vi "VI CAN Konfig.vi"() -> ()   [LabVIEW 2020, in "CAN Konfig.lvlib"]
uses:
  CAN Konfig.lvlib
  Konfig Daten PC.ctl
  cRIO/CAN Interface/Baude Rate.ctl
  Visualisierungs Elemente/Button.ctl
  Aktion FGV CAN.ctl
  FT-IR/FGV FT-IR Gasliste Aktionen.ctl
  Passwortverwaltung/FGV Passwort Aktion.ctl
  Aktion Tabellen ziehen.ctl
  Allgemein/Aktionen Daten am cRIO speichern.ctl
  FT-IR/FGV FT-IR Aktionen.ctl
  SysLog/SysLog Interface.ctl
  Visualisierungs Elemente/String - Ausgabefeld.ctl
  Allgemein/allgemeine Sub-VIs.lvlib
  FT-IR/FT-IR.lvlib
  Sprachverwaltung/Sprachverwaltung.lvlib
  SysLog/SysLog.lvlib
  Passwortverwaltung/Passwort.lvlib
  cRIO/CAN Interface/CAN Interface.lvlib
panel:
  in  "exportieren":T1 caption="speichern"
  out "Status":u32[](array[numeric])
  in  "laden":T1 caption="speichern"
  in  "Konfig Daten":T2={"Baude Rate"=250000, "COM state"=0, "Frame-ID FTIR Start"=0, "Frame-ID FTIR End"=0, "Frame-ID Status Start"=0, "Frame-ID Status End"=0, "Zustand Information"=0, "Aktion"=0, "Frame-ID FTIR Arry"=[], "Frame-ID Status Arry"=[], "GPS Start"=0, "Interface"="CAN1"} {"Baude Rate" items=["40 kBaud"=40000, "50 kBaud"=50000, "62,5 kBaud"=62500, "80 kBaud"=80000, "83,3 kBaud"=83300, "100 kBaud"=100000, "125 kBaud"=125000, "160 kBaud"=160000, "200 kBaud"=200000, "250 kBaud"=250000, "400 kBaud"=400000, "500 kBaud"=500000, "800 kBaud"=800000, "1 MBaud"=1000000]}
  in  "Optionsfelder FT-IR":T4(radio)
  in  "Optionsfelder Status":T4(radio)
  in  "Tabellenelement FT-IR":string[][](table)
  in  "Tabellenelement Status":string[][](table)
  in  "Löschen Status":bool
  in  "Entfernen Status":bool
  in  "Hinzufügen Status":bool
  in  "Konfigurierte Liste Status":i32(listbox)=-1 caption="Konfigurierte Liste"
  in  "Statusliste":i32(listbox)=-1 caption="Original Liste"
  in  "Löschen FTIR 1":bool
  in  "Entfernen FTIR 1":bool
  in  "Hinzufügen FTIR 1":bool
  in  "speichern":T1
  in  "Konfigurierte Liste 1":i32(listbox)=-1 caption="Konfigurierte Liste"
  in  "Original Liste":i32(listbox)=-1
  in  "apply":T1 caption="speichern"
  # "CAN Config"
  # "Scale"
  # "Scale"
  # "CAN Parameter"
  # "Status Frame"
  # "Status Value"
  # "FTIR Frame"
  # "Gaslist"
  # "CAN Measurement Data"
  # "CAN Status Value"
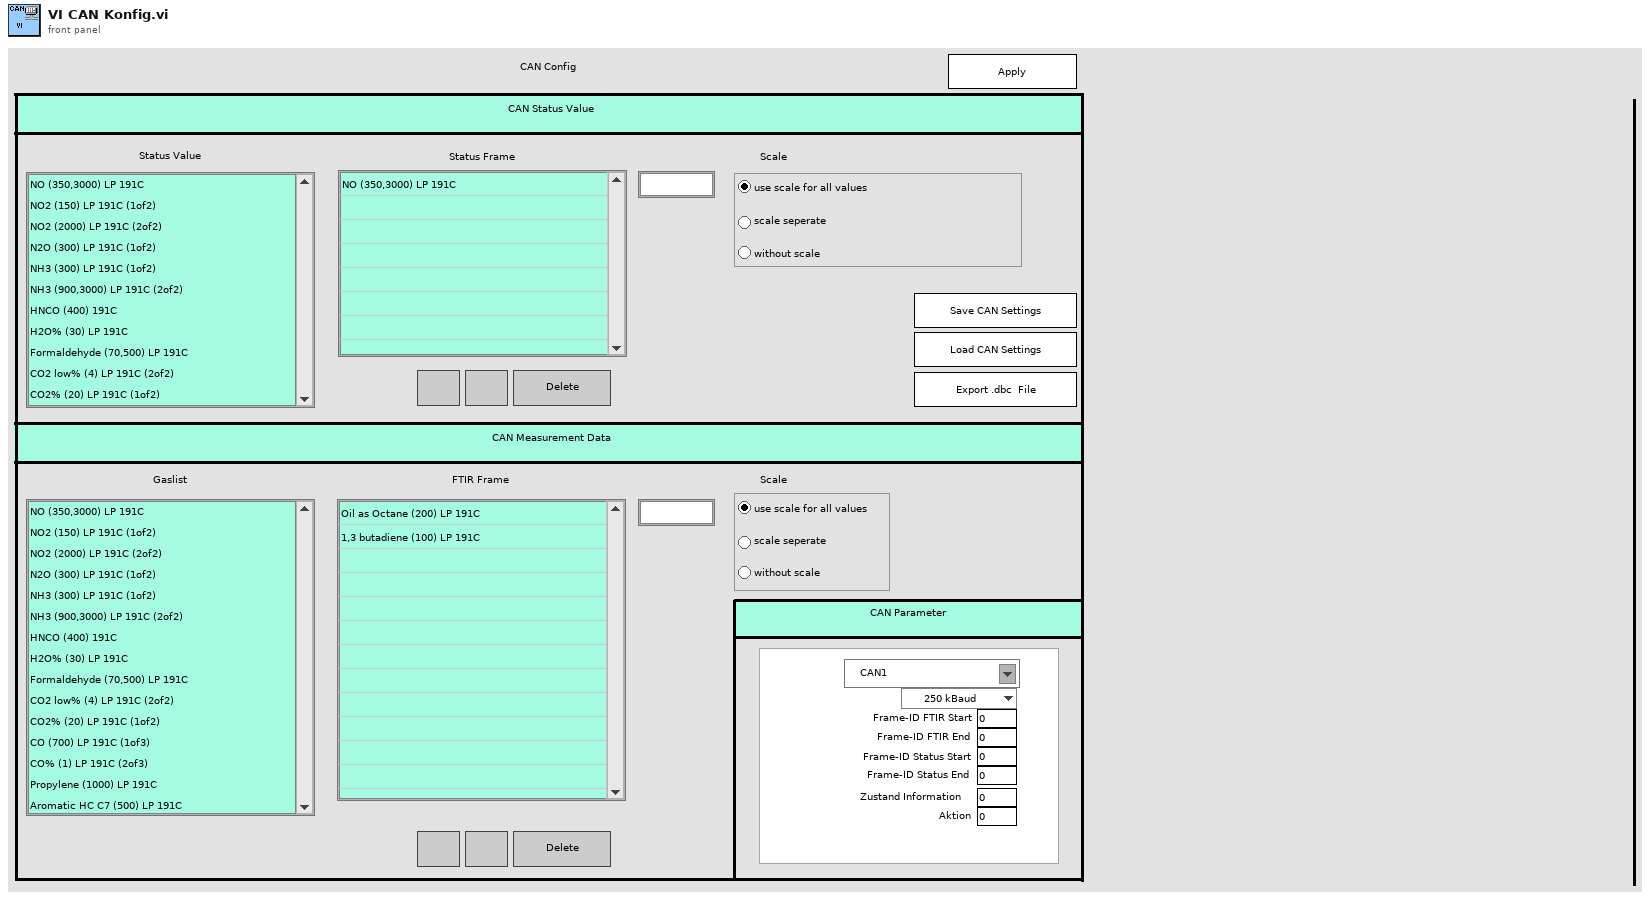
[diagram p1: front panel]
types:
  T1 = typedef "Button.ctl" = bool
  T2 = typedef "CAN Konfig.lvlib/Konfig Daten PC.ctl" = cluster{"Baude Rate":T3, "COM state":u8, "Frame-ID FTIR Start":u32, "Frame-ID FTIR End":u32, "Frame-ID Status Start":u32, "Frame-ID Status End":u32, "Zustand Information":u32, "Aktion":u32, "Frame-ID FTIR Arry":u32[], "Frame-ID Status Arry":u32[], "GPS Start":u32, "Interface":refnum<k21>}
  T3 = typedef "CAN Interface.lvlib/Baude Rate.ctl" = u32
  T4 = enum32{"Optionsauswahl 1", "Optionsauswahl 2", "Optionsauswahl 3"}
  T5 = typedef "Passwort.lvlib/FGV Passwort Aktion.ctl" = enum16{"prüfen", "setzen", "Initialisieren", "PW speichern", "lesen", "PW Änderung"}
  T6 = typedef "FT-IR.lvlib/FGV FT-IR Gasliste Aktionen.ctl" = enum16{"lesen", "Gasliste FT-IR", "Gasliste ausgelesen", "laden", "speichern", "löschen"}
  T7 = typedef "CAN Konfig.lvlib/Aktion FGV CAN.ctl" = enum16{"lesen", "schreiben Konfig", "Status", "Messdaten", "laden", "speichern", "CAN Data"}
  T8 = typedef "CAN Konfig.lvlib/Aktion Tabellen ziehen.ctl" = enum16{"ini", "prüfen"}
  T9 = typedef "CAN Konfig.lvlib/CAN Messdaten.ctl" = cluster{"FTIR 1 Index":i32[], "FTIR 2 Index":i32[], "Status Index":i32[], "FT-IR Scale":sgl[], "Status Scale":sgl[], "Optionsfelder FT-IR":enum32{"Optionsauswahl 1", "Optionsauswahl 2", "Optionsauswahl 3"}, "Optionsfelder Status":enum32{"Optionsauswahl 1", "Optionsauswahl 2", "Optionsauswahl 3"}}
  T10 = typedef "String - Ausgabefeld.ctl" = string
  T11 = typedef "allgemeine Sub-VIs.lvlib/Aktionen Daten am cRIO speichern.ctl" = enum16{"lesen", "speichern setzen", "speichern reset", "gespeichert"}
  T12 = typedef "FT-IR.lvlib/FGV FT-IR Aktionen.ctl" = enum16{"lesen", "NOG setzen", "NOS setzen", "Initialisieren", "speichern", "ALLES setzen", "FT-IR Spektrum loggen", "Komm Stoppen", "Spektrum LogKonfig"}
  T13 = typedef "SysLog.lvlib/SysLog Interface.ctl" = cluster{"FehlermeldungsCode":i32, "ErfolgsmeldungsCode":i32, "ParameterListenString":string, "Anzeige":bool, "SysLogIcon":enum16{"OK", "Warnung", "Fehler"}, "intern":bool}
  T14 = enum16{"Left Button", "Center Button", "Right Button", "Window Close"}
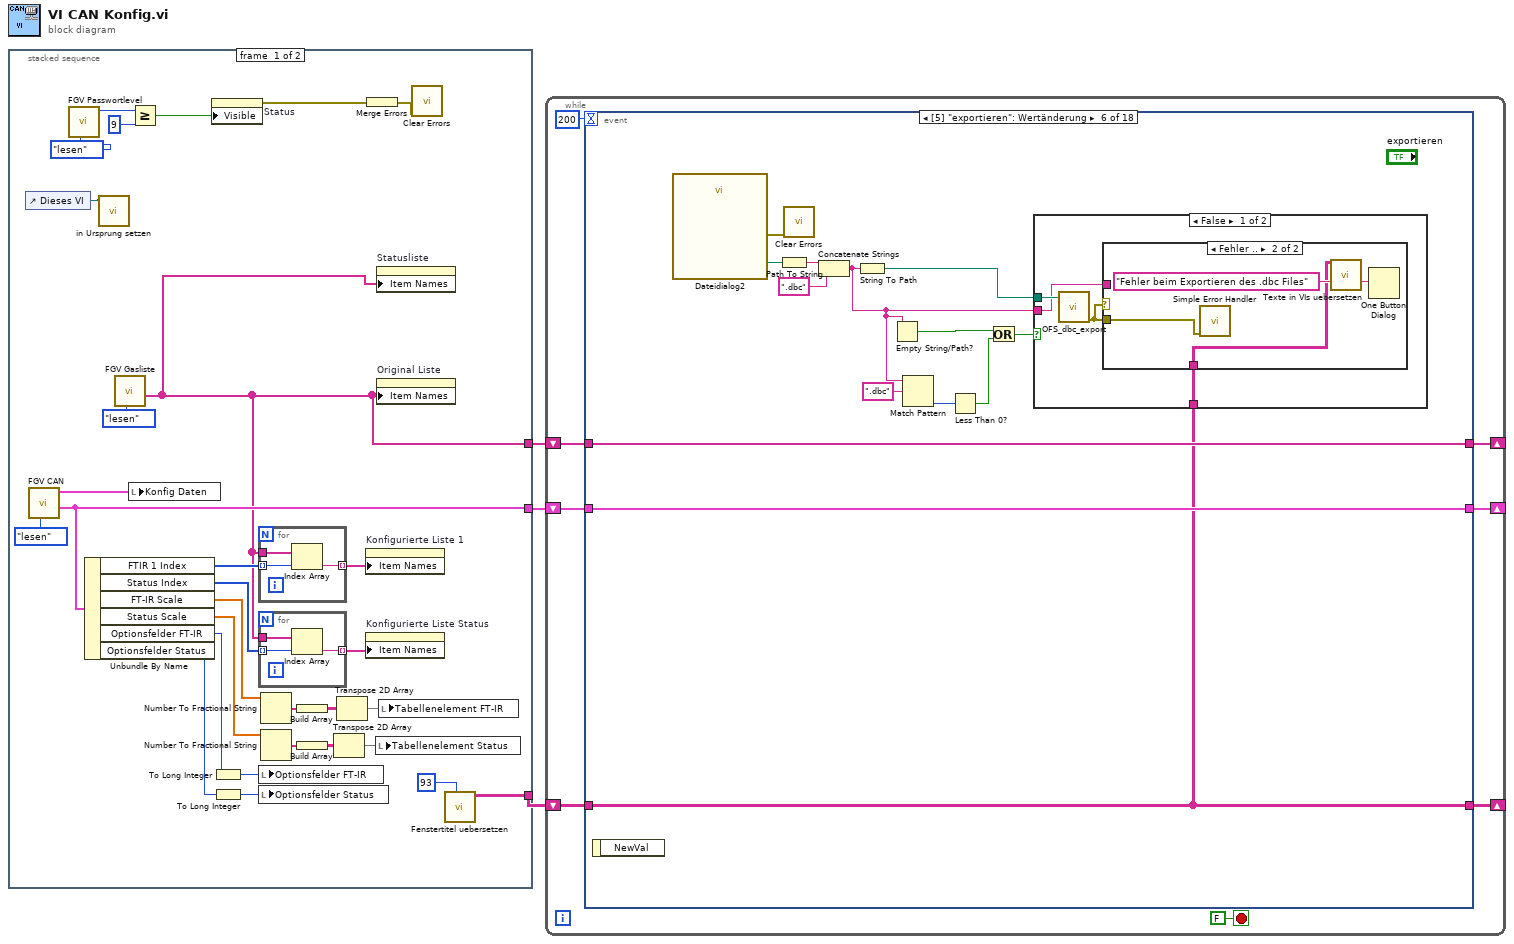
[diagram p0: block diagram]
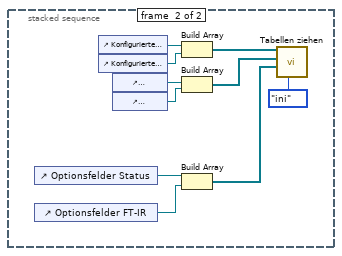
[diagram p2: hidden frame]
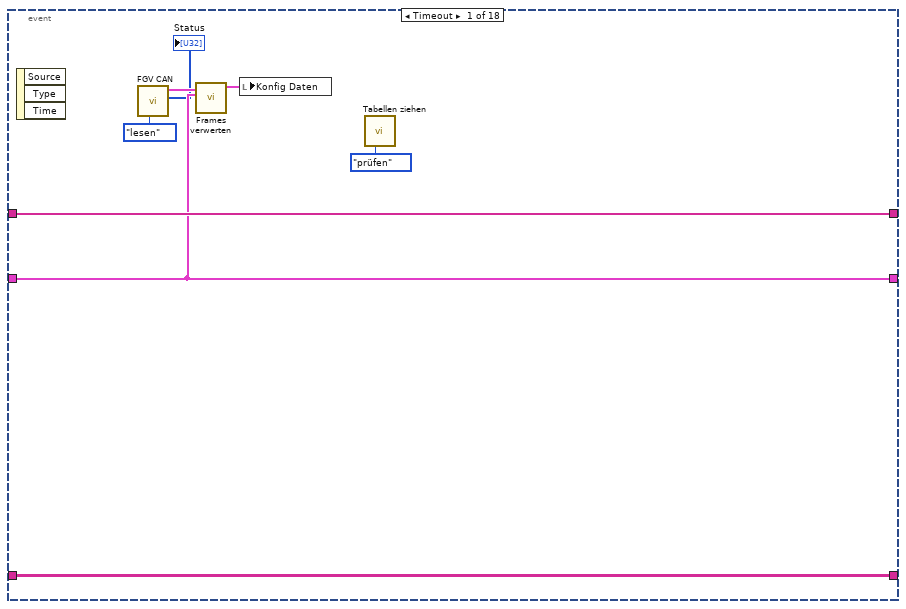
[diagram p3: hidden frame]
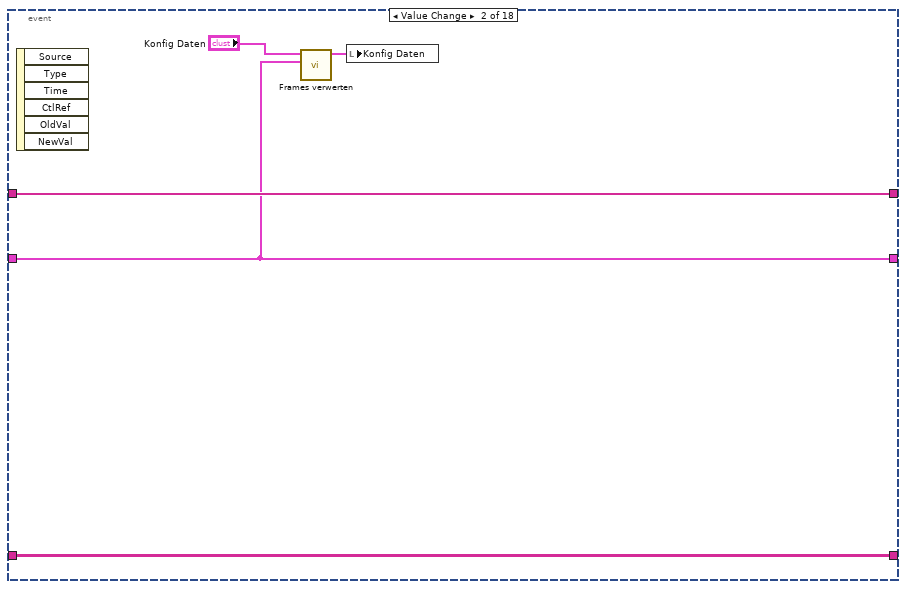
[diagram p4: hidden frame]
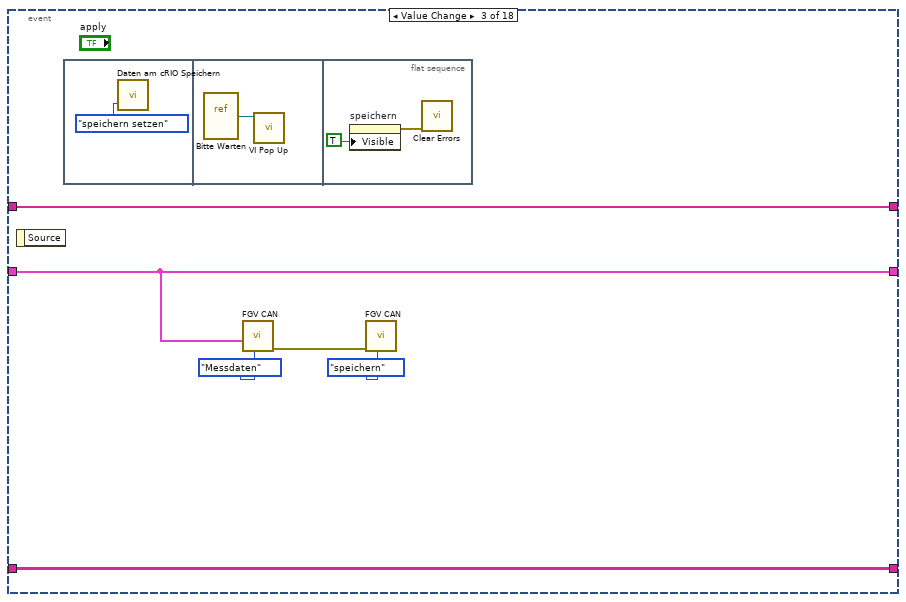
[diagram p5: hidden frame]
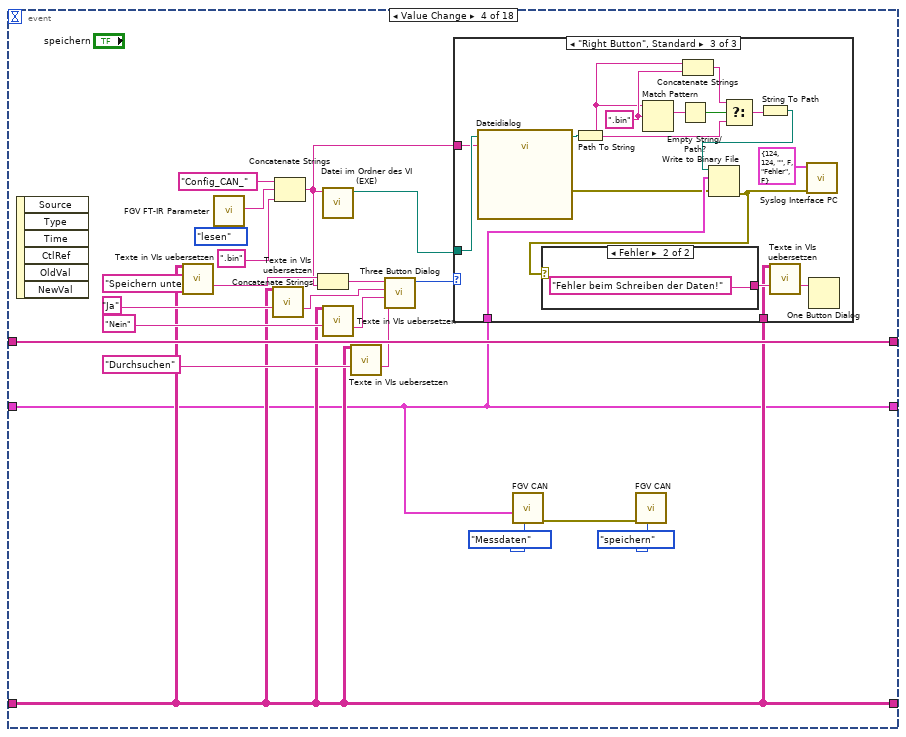
[diagram p6: hidden frame]
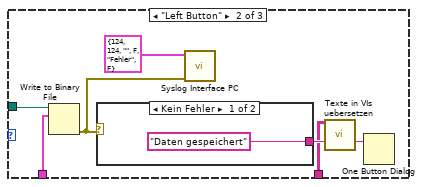
[diagram p8: hidden frame]
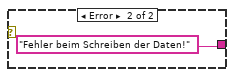
[diagram p9: hidden frame]
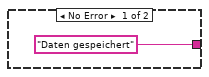
[diagram p10: hidden frame]
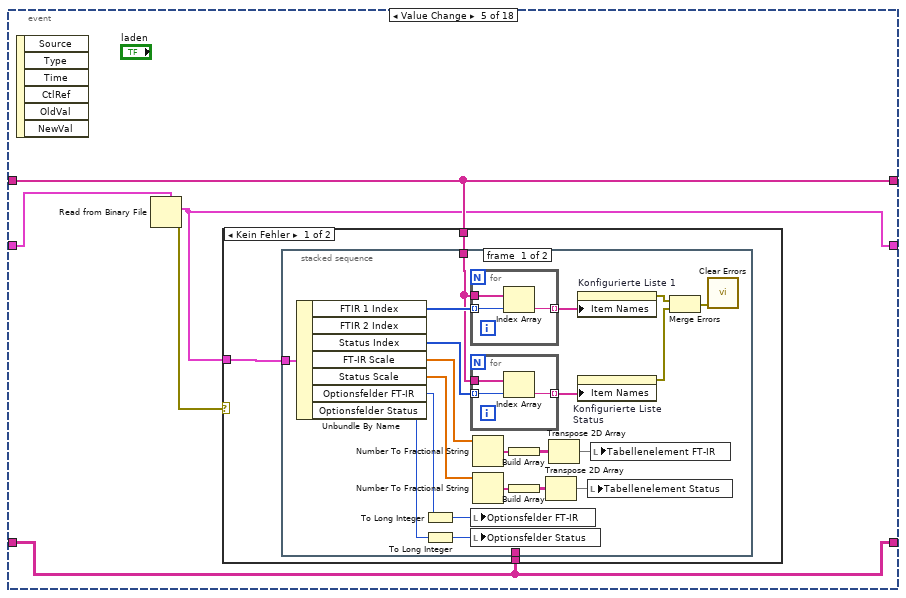
[diagram p11: hidden frame]
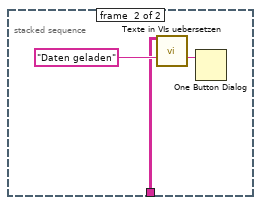
[diagram p12: hidden frame]
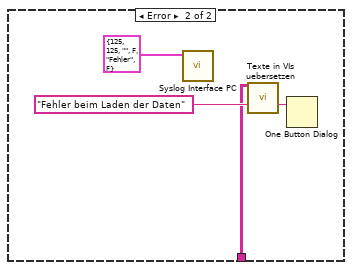
[diagram p13: hidden frame]
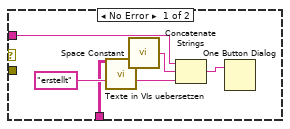
[diagram p14: hidden frame]
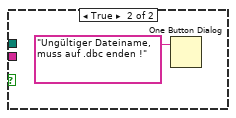
[diagram p15: hidden frame]
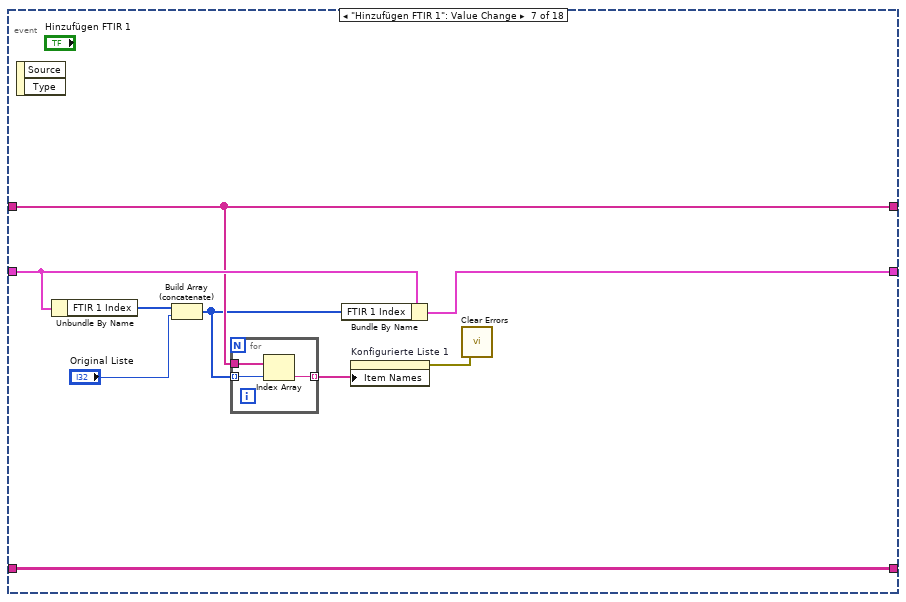
[diagram p16: hidden frame]
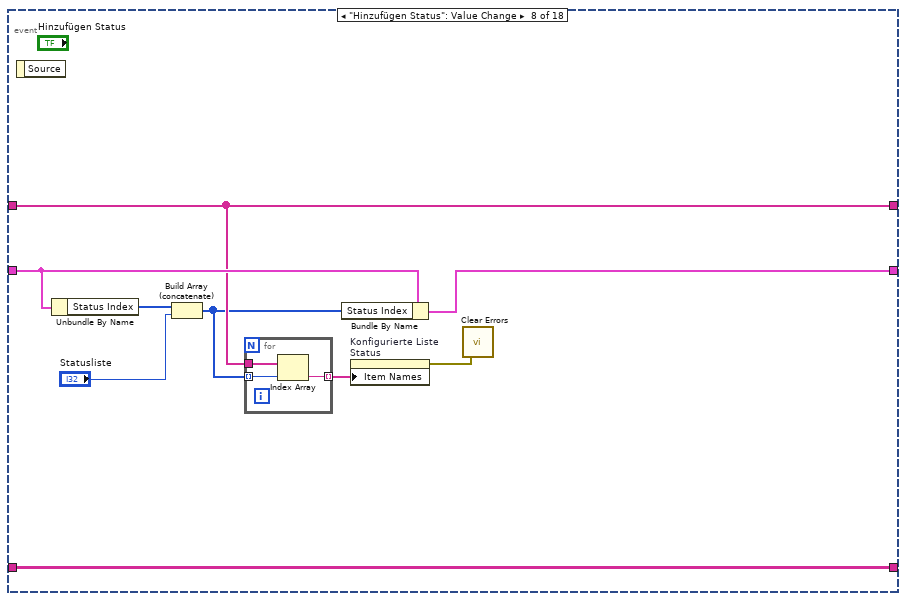
[diagram p17: hidden frame]
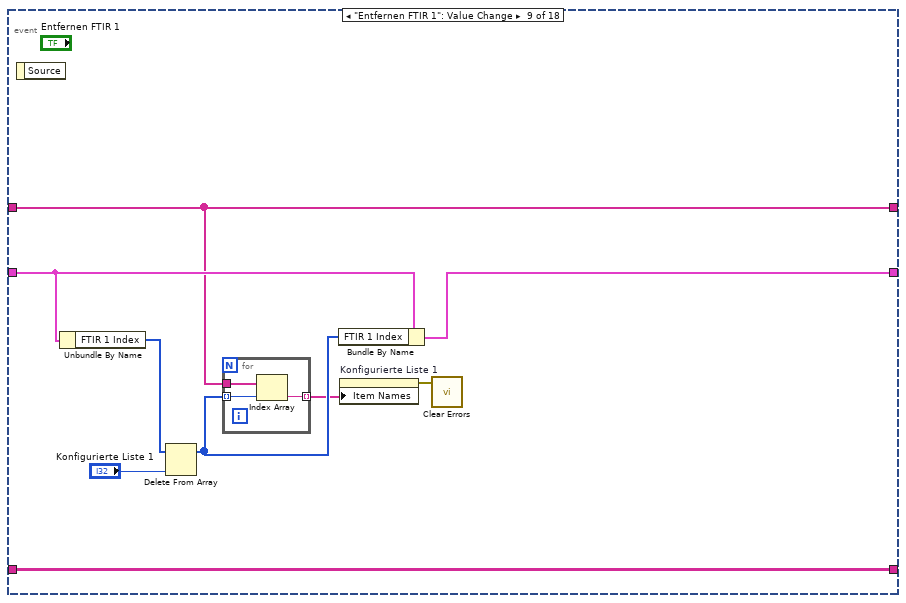
[diagram p18: hidden frame]
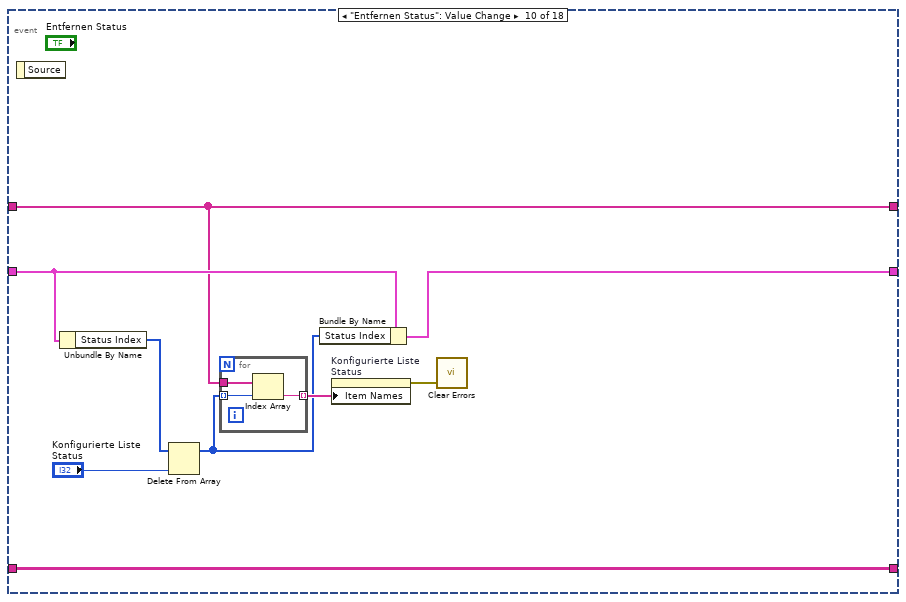
[diagram p19: hidden frame]
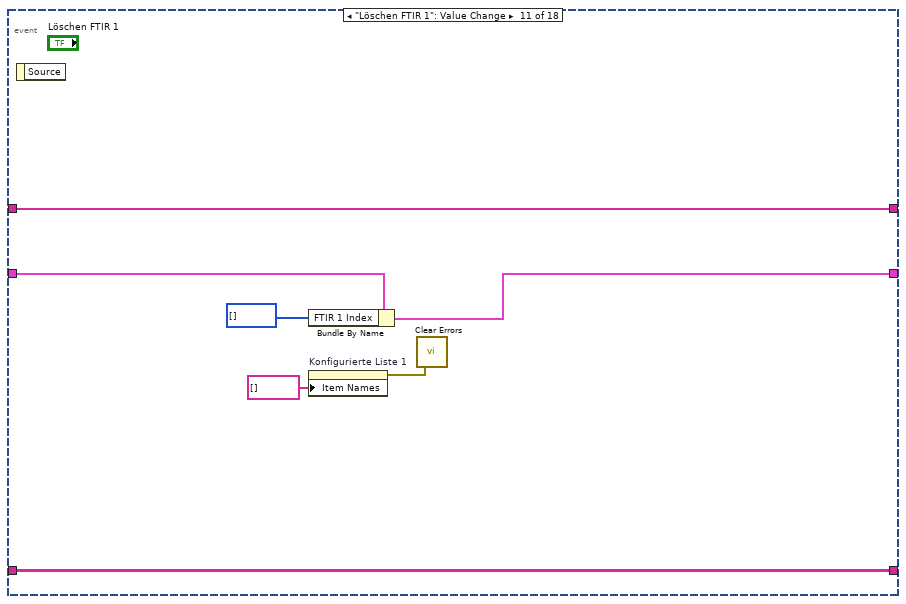
[diagram p20: hidden frame]
diagram:
  n1 = stacked-sequence {
    tunnel: [w4 _] -> w3
    tunnel: [w29 _] -> w2
    tunnel: [w11 _] -> w1
    frame #0 {
      n2 = control-ref of="Dieses VI"() -> (w25:refnum<vi>)
      n3 = call "FGV CAN.vi"("Aktion"=Aktion_FGV_CAN."lesen") -> ("CAN Messdaten"=w29:T9, "Konfig Daten"=w32:T2)  [unwired: 6 in, 3 out]
      n4 = call "FGV Passwortlevel.vi"("FGV Passwort Aktion"=FGV_Passwort_Aktion."lesen") -> ("aktueller Level"=w8:i16)  [unwired: 8 in, 2 out]
      n5 = Unbundle By Name(w29) -> ("FTIR 1 Index"=w30:i32[], "Status Index"=w27:i32[], "FT-IR Scale"=w24:sgl[], "Status Scale"=w23:sgl[], "Optionsfelder FT-IR"=w18:T4, "Optionsfelder Status"=w16:T4)
      n6 = call "in Ursprung setzen.vi"("VI Referenz"=w25) -> ()  [unwired: 10 in, 1 out]
      n7 = call "FGV Gasliste.vi"("Aktionen"=FGV_FT-IR_Gasliste_Aktionen."lesen") -> ("Aktuelle Gasliste gesamt"=w4:T10[])  [unwired: 8 in, 2 out]
      n8 = local write "Konfig Daten"(w32) -> ()
      n9 = Greater Or Equal?(x=w8, y=i16 9 ("x")) -> (x >= y?=w7:bool)
      n10 = property on="Status" class="Arr (strikt)"("Visible"=w7) -> (error out=w6:errorcluster)  [unwired: 2 in, 1 out]
      n11 = To Long Integer(number=w18) -> (32bit integer=w17:i32)
      n12 = To Long Integer(number=w16) -> (32bit integer=w15:i32)
      n13 = for {
        tunnel: w30 -> [w39] mode=indexing
        tunnel: w4 -> [w38]
        tunnel: [w37] -> w31 mode=indexing
        n14 = Index Array(array=w38, index=w39) -> (element=w37:T10)
      }
      n15 = for {
        tunnel: [w36] -> w28 mode=indexing
        tunnel: w27 -> [w35] mode=indexing
        tunnel: w4 -> [w34]
        n16 = Index Array(array=w34, index=w35) -> (element=w36:T10)
      }
      n17 = local write "Optionsfelder FT-IR"(w17) -> ()
      n18 = local write "Optionsfelder Status"(w15) -> ()
      n19 = Number To Fractional String(number=w24) -> (F-format string=w19:string[])  [unwired: 3 in]
      n20 = Number To Fractional String(number=w23) -> (F-format string=w22:string[])  [unwired: 3 in]
      n21 = Build Array(w19) -> (w20:string[][])
      n22 = Build Array(w22) -> (w21:string[][])
      n23 = Transpose 2D Array(2D array=w21) -> (transposed array=w13:string[][])
      n24 = Transpose 2D Array(2D array=w20) -> (transposed array=w14:string[][])
      n25 = property on="Konfigurierte Liste 1" class="Listenfeld (strikt)"("Item Names"=w31) -> ()  [unwired: 2 in, 2 out]
      n26 = property on="Konfigurierte Liste Status" class="Listenfeld (strikt)"("Item Names"=w28) -> ()  [unwired: 2 in, 2 out]
      n27 = Merge Errors(w6) -> (w5:errorcluster)
      n28 = local write "Tabellenelement Status"(w13) -> ()
      n29 = property on="Statusliste" class="Listenfeld (strikt)"("Item Names"=w4) -> ()  [unwired: 2 in, 2 out]
      n30 = property on="Original Liste" class="Listenfeld (strikt)"("Item Names"=w4) -> ()  [unwired: 2 in, 2 out]
      n31 = local write "Tabellenelement FT-IR"(w14) -> ()
      n32 = call <vilib>:"Clear Errors.vi"("error in (no error)"=w5) -> ()  [unwired: 5 in, 2 out]
      n33 = call "Fenstertitel uebersetzen.vi"("Index (Seite)"=93) -> ("Sprachliste"=w11:string[][])  [unwired: 7 in, 3 out]
    }
    frame #1 {
      n34 = control-ref of="Optionsfelder Status"() -> (w43:refnum<vi>)
      n35 = control-ref of="Optionsfelder FT-IR"() -> (w42:refnum<vi>)
      n36 = control-ref of="Konfigurierte Liste Status"() -> (w46:refnum<vi>)
      n37 = control-ref of="Konfigurierte Liste 1"() -> (w47:refnum<vi>)
      n38 = control-ref of="Tabellenelement Status"() -> (w48:refnum<vi>)
      n39 = control-ref of="Tabellenelement FT-IR"() -> (w49:refnum<vi>)
      n40 = Build Array(w46, w47) -> (w45:refnum<vi>[])
      n41 = Build Array(w48, w49) -> (w44:refnum<vi>[])
      n42 = Build Array(w43, w42) -> (w41:refnum<vi>[])
      n43 = call "Tabellen ziehen.vi"("Aktion"=Aktion_Tabellen_ziehen."ini", "Angehängtes Array"=w41, "Tabelle (Eingang)"=w44, "Konfigurierte Liste Status"=w45) -> ()  [unwired: 8 in]
    }
  }
  n44 = while {
    shift-right: [w55] -> _
    shift-left: w3 -> [w56]
    shift-right: [w53] -> _
    shift-left: w2 -> [w54]
    shift-right: [w50] -> _
    shift-left: w1 -> [w51]
    stop <- FALSE stop-if-true
    n45 = event shown="[5] \"exportieren\": Wertänderung" {
      selector: _ -> [_ _ _ _ _ _ _ _ _ _ _ _ _ _ _ _ _ _]
      dyn-events: _ -> [_ _ _ _ _ _ _ _ _ _ _ _ _ _ _ _ _ _]
      timeout: 200 -> [_ _ _ _ _ _ _ _ _ _ _ _ _ _ _ _ _ _]
      tunnel: w56 -> [w65 w70 w76 w102 w135 w186 w204 w215 w227 w239 w256 w263 w274 w304 w333 w343 w349 w360]
      tunnel: [w65 w70 w76 w102 w135 w186 w204 w215 w227 w239 w256 w263 w274 w304 w333 w343 w349 w360] -> w55
      tunnel: w54 -> [w61 w68 w72 w81 w134 w185 w209 w221 w234 w246 w255 w262 w270 w300 w327 w337 w348 w359]
      tunnel: [w61 w68 w72 w81 w133 w185 w208 w220 w231 w244 w254 w261 w273 w303 w325 w335 w345 w356] -> w53
      tunnel: w51 -> [w59 w66 w71 w87 w131 w173 w206 w217 w229 w241 w251 w257 w264 w294 w324 w334 w344 w355]
      tunnel: [w59 w66 w71 w87 w131 w173 w206 w217 w229 w241 w251 w257 w264 w294 w324 w334 w344 w355] -> w50
      event Timeout {
        n46 = event-data() -> ()  [unwired: 1 in, 3 out]
        n47 = call "FGV CAN.vi"("Aktion"=Aktion_FGV_CAN."lesen") -> ("Status"=→"Status":u32[], "Konfig Daten"=w62:T2)  [unwired: 6 in, 3 out]
        n48 = call "Frames verwerten.vi"("CAN Messdaten"=w61, "Konfig Daten"=w62) -> ("Ausgangs-Cluster"=w63:T2)  [unwired: 9 in]
        n49 = local write "Konfig Daten"(w63) -> ()
        n50 = call "Tabellen ziehen.vi"("Aktion"=Aktion_Tabellen_ziehen."prüfen") -> ()  [unwired: 11 in]
      }
      event Value Change {
        n51 = event-data() -> ()  [unwired: 1 in, 6 out]
        n52 = call "Frames verwerten.vi"("CAN Messdaten"=w68, "Konfig Daten"="Konfig Daten") -> ("Ausgangs-Cluster"=w67:T2)  [unwired: 9 in]
        n53 = local write "Konfig Daten"(w67) -> ()
      }
      event Value Change {
        n54 = event-data() -> ()  [unwired: 1 in, 1 out]
        n55 = flat-sequence {
          frame #0 {
            n56 = call "Daten am cRIO Speichern.vi"("Aktionen"=Aktionen_Daten_am_cRIO_speichern."speichern setzen") -> ()  [unwired: 9 in, 2 out]
          }
          frame #1 {
            n57 = vi-ref "Bitte Warten.vi"() -> (w78:refnum<vi>)
            n58 = call "VI Pop Up.vi"("VI Referenz"=w78) -> ()  [unwired: 10 in, 1 out]
          }
          frame #2 {
            n59 = property on="speichern" class="Bool."("Visible"=TRUE ("Sichtbar")) -> (error out=w79:errorcluster)  [unwired: 2 in, 1 out]
            n60 = call <vilib>:"Clear Errors.vi"("error in (no error)"=w79) -> ()  [unwired: 5 in, 2 out]
          }
        }
        n61 = call "FGV CAN.vi"("Aktion"=Aktion_FGV_CAN."Messdaten", "CAN Messdaten"=w72) -> ("error out"=w73:errorcluster)  [unwired: 5 in, 4 out]
        n62 = call "FGV CAN.vi"("Aktion"=Aktion_FGV_CAN."speichern", "error in (no error)"=w73) -> ()  [unwired: 5 in, 5 out]
      }
      event Value Change {
        n63 = event-data() -> ()  [unwired: 1 in, 6 out]
        n64 = call "Texte in VIs uebersetzen.vi"("Sprachliste"=w87, "String zum Übersetzen"="Speichern unter ") -> ("String zum Übersetzen"=w91:string)  [unwired: 9 in, 4 out]
        n65 = call "FGV FT-IR Parameter.vi"("Aktion"=FGV_FT-IR_Aktionen."lesen") -> ("Current Recipe"=w99:string)  [unwired: 11 in, 7 out]
        n66 = call "Texte in VIs uebersetzen.vi"("Sprachliste"=w87, "String zum Übersetzen"="Ja") -> ("String zum Übersetzen"=w90:string)  [unwired: 9 in, 4 out]
        n67 = Concatenate Strings("Config_CAN_" ("Dateiname"), w99, ".bin" ("Dateiname")) -> (w85:string)
        n68 = Concatenate Strings(w91, w85) -> (w96:string)
        n69 = call "Datei im Ordner des VI (EXE).vi"("Dateiname"=w85) -> ("Dateipfad im Ordner des Haupt-VIs"=w97:path)  [unwired: 8 in, 2 out]
        n70 = call "Texte in VIs uebersetzen.vi"("Sprachliste"=w87, "String zum Übersetzen"="Nein") -> ("String zum Übersetzen"=w89:string)  [unwired: 9 in, 4 out]
        n71 = call "Texte in VIs uebersetzen.vi"("Sprachliste"=w87, "String zum Übersetzen"="Durchsuchen") -> ("String zum Übersetzen"=w86:string)  [unwired: 9 in, 4 out]
        n72 = call <vilib>:"Three Button Dialog.vi"("Right Button Text (\"Cancel\")"=w86, "Center Button Text (\"No\")"=w89, "Left Button Text (\"Yes\")"=w90, "message"=w96) -> ("Which Button?"=w95:T14)  [unwired: 7 in]
        n73 = case shown="\"Right Button\", Standard" w95 {
          tunnel: w97 -> [_ w109 w125]
          tunnel: w81 -> [_ w108 w123]
          tunnel: w87 -> [_ w105 w126]
          tunnel: w85 -> [_ _ w124]
          frame "Center Button" {
          }
          frame "Left Button" {
            n74 = Write to Binary File(file (use dialog)=w109, data=w108) -> (error out=w103:errorcluster)  [unwired: 1 in, 5 out]
            n75 = case shown="Kein Fehler" w103 {
              tunnel: ["Daten gespeichert" ("String") "Fehler beim Schreiben der Daten!" ("String")] -> w107
              frame No Error {
              }
              frame Error {
              }
            }
            n76 = call "Syslog Interface PC.vi"("Fehler (in)"=w103, "Cluster (in)"=T13 {"FehlermeldungsCode"=124, "ErfolgsmeldungsCode"=124, "ParameterListenString"="", "Anzeige"=FALSE, "SysLogIcon"=enum."Fehler", "intern"=FALSE}) -> ()  [unwired: 9 in, 1 out]
            n77 = call "Texte in VIs uebersetzen.vi"("Sprachliste"=w105, "String zum Übersetzen"=w107) -> ("String zum Übersetzen"=w106:string)  [unwired: 9 in, 4 out]
            n78 = One Button Dialog(message=w106) -> ()  [unwired: 1 in, 1 out]
          }
          frame "Right Button", Default {
            w115 = ".bin" ("Regulärer Ausdruck")
            n79 = call "Dateidialog"("start path"=w125, "default name"=w124) -> ("selected path"=w120:path, "error out"=w118:errorcluster)  [unwired: 10 in, 2 out]
            n80 = Path To String(path=w120) -> (string=w113:string)
            n81 = Match Pattern(string=w113, regular expression=w115) -> (match substring=w116:string)  [unwired: 1 in, 3 out]
            n82 = Empty String/Path?(string/path=w116) -> (empty?=w117:bool)
            n83 = Concatenate Strings(w113, w115) -> (w114:string)
            n84 = Select(t=w114, s=w117, f=w113) -> (s? t:f=w112:string)
            n85 = String To Path(string=w112) -> (path=w119:path)
            n86 = Write to Binary File(file (use dialog)=w119, data=w123, error in=w118) -> (error out=w121:errorcluster)  [unwired: 5 out]
            n87 = case shown="Fehler" w121 {
              tunnel: ["Daten gespeichert" ("String") "Fehler beim Schreiben der Daten!" ("String")] -> w128
              frame No Error {
              }
              frame Error {
              }
            }
            n88 = call "Texte in VIs uebersetzen.vi"("Sprachliste"=w126, "String zum Übersetzen"=w128) -> ("String zum Übersetzen"=w127:string)  [unwired: 9 in, 4 out]
            n89 = call "Syslog Interface PC.vi"("Fehler (in)"=w121, "Cluster (in)"=T13 {"FehlermeldungsCode"=124, "ErfolgsmeldungsCode"=124, "ParameterListenString"="", "Anzeige"=FALSE, "SysLogIcon"=enum."Fehler", "intern"=FALSE}) -> ()  [unwired: 9 in, 1 out]
            n90 = One Button Dialog(message=w127) -> ()  [unwired: 1 in, 1 out]
          }
        }
        n91 = call "FGV CAN.vi"("Aktion"=Aktion_FGV_CAN."Messdaten", "CAN Messdaten"=w81) -> ("error out"=w82:errorcluster)  [unwired: 5 in, 4 out]
        n92 = call "FGV CAN.vi"("Aktion"=Aktion_FGV_CAN."speichern", "error in (no error)"=w82) -> ()  [unwired: 5 in, 5 out]
      }
      event Value Change {
        n93 = event-data() -> ()  [unwired: 1 in, 6 out]
        n94 = Read from Binary File(5:w134) -> (0:w132:errorcluster, 2:w133:T9)  [unwired: 2 in, 5 out]
        n95 = case shown="Kein Fehler" w132 {
          tunnel: w135 -> [w138 _]
          tunnel: w133 -> [w137 _]
          tunnel: w131 -> [w136 w170]
          frame No Error {
            n96 = stacked-sequence {
              tunnel: w138 -> [w143 _]
              tunnel: w137 -> [w142 _]
              tunnel: w136 -> [_ w166]
              frame #0 {
                n97 = Unbundle By Name(w142) -> ("FTIR 1 Index"=w145:i32[], "Status Index"=w147:i32[], "FT-IR Scale"=w148:sgl[], "Status Scale"=w149:sgl[], "Optionsfelder FT-IR"=w154:T4, "Optionsfelder Status"=w156:T4)  [unwired: 1 out]
                n98 = To Long Integer(number=w154) -> (32bit integer=w155:i32)
                n99 = To Long Integer(number=w156) -> (32bit integer=w157:i32)
                n100 = for {
                  tunnel: w145 -> [w165] mode=indexing
                  tunnel: w143 -> [w164]
                  tunnel: [w163] -> w144 mode=indexing
                  n101 = Index Array(array=w164, index=w165) -> (element=w163:T10)
                }
                n102 = for {
                  tunnel: [w162] -> w146 mode=indexing
                  tunnel: w147 -> [w161] mode=indexing
                  tunnel: w143 -> [w160]
                  n103 = Index Array(array=w160, index=w161) -> (element=w162:T10)
                }
                n104 = local write "Optionsfelder FT-IR"(w155) -> ()
                n105 = local write "Optionsfelder Status"(w157) -> ()
                n106 = Number To Fractional String(number=w148) -> (F-format string=w153:string[])  [unwired: 3 in]
                n107 = Number To Fractional String(number=w149) -> (F-format string=w150:string[])  [unwired: 3 in]
                n108 = Build Array(w153) -> (w152:string[][])
                n109 = Build Array(w150) -> (w151:string[][])
                n110 = Transpose 2D Array(2D array=w151) -> (transposed array=w159:string[][])
                n111 = Transpose 2D Array(2D array=w152) -> (transposed array=w158:string[][])
                n112 = property on="Konfigurierte Liste 1" class="Listenfeld (strikt)"("Item Names"=w144) -> (error out=w140:errorcluster)  [unwired: 2 in, 1 out]
                n113 = property on="Konfigurierte Liste Status" class="Listenfeld (strikt)"("Item Names"=w146) -> (error out=w139:errorcluster)  [unwired: 2 in, 1 out]
                n114 = local write "Tabellenelement Status"(w159) -> ()
                n115 = local write "Tabellenelement FT-IR"(w158) -> ()
                n116 = Merge Errors(w140, w139) -> (w141:errorcluster)
                n117 = call <vilib>:"Clear Errors.vi"("error in (no error)"=w141) -> ()  [unwired: 5 in, 2 out]
              }
              frame #1 {
                n118 = call "Texte in VIs uebersetzen.vi"("Sprachliste"=w166, "String zum Übersetzen"="Daten geladen" ("String")) -> ("String zum Übersetzen"=w168:string)  [unwired: 9 in, 4 out]
                n119 = One Button Dialog(message=w168) -> ()  [unwired: 1 in, 1 out]
              }
            }
          }
          frame Error {
            n120 = call "Syslog Interface PC.vi"("Cluster (in)"=T13 {"FehlermeldungsCode"=125, "ErfolgsmeldungsCode"=125, "ParameterListenString"="", "Anzeige"=FALSE, "SysLogIcon"=enum."Fehler", "intern"=FALSE}) -> ()  [unwired: 10 in, 1 out]
            n121 = call "Texte in VIs uebersetzen.vi"("Sprachliste"=w170, "String zum Übersetzen"="Fehler beim Laden der Daten" ("String")) -> ("String zum Übersetzen"=w172:string)  [unwired: 9 in, 4 out]
            n122 = One Button Dialog(message=w172) -> ()  [unwired: 1 in, 1 out]
          }
        }
      }
      event Value Change {
        n123 = event-data() -> ()  [unwired: 1 in, 1 out]
        n124 = call "Dateidialog2"() -> ("selected path"=w179:path, "error out"=w174:errorcluster)  [unwired: 12 in, 2 out]
        n125 = Path To String(path=w179) -> (string=w178:string)
        n126 = call <vilib>:"Clear Errors.vi"("error in (no error)"=w174) -> ()  [unwired: 5 in, 2 out]
        n127 = Concatenate Strings(w178, ".dbc" ("String")) -> (w175:string)
        n128 = String To Path(string=w175) -> (path=w176:path)
        n129 = Empty String/Path?(string/path=w175) -> (empty?=w182:bool)
        n130 = Match Pattern(string=w175, regular expression=".dbc" ("Regulärer Ausdruck")) -> (offset past match=w183:i32)  [unwired: 1 in, 3 out]
        n131 = Less Than 0?(x=w183) -> (x < 0?=w181:bool)
        n132 = Or(x=w182, y=w181) -> (x .or. y?=w180:bool)
        n133 = case shown="False" w180 {
          tunnel: w176 -> [w190 _]
          tunnel: w175 -> [w189 _]
          tunnel: w173 -> [w187 _]
          frame False {
            n134 = call "OFS_dbc_export.vi"(".dbc File"=w190) -> ("Fehler (Ausgang)"=w188:errorcluster)  [unwired: 10 in]
            n135 = case shown="Fehler .." w188 {
              tunnel: w188 -> [_ w200]
              tunnel: w189 -> [w195 _]
              tunnel: w187 -> [w191 w197]
              frame No Error {
                n136 = call "Texte in VIs uebersetzen.vi"("Sprachliste"=w191, "String zum Übersetzen"="erstellt" ("String")) -> ("String zum Übersetzen"=w192:string)  [unwired: 9 in, 4 out]
                n137 = call <vilib>:"Space Constant.vi"() -> ("String"=w194:string)
                n138 = Concatenate Strings(w195, w194, w192) -> (w196:string)
                n139 = One Button Dialog(message=w196) -> ()  [unwired: 1 in, 1 out]
              }
              frame Error {
                n140 = call <vilib>:"Simple Error Handler.vi"("error in (no error)"=w200) -> ()  [unwired: 4 in, 5 out]
                n141 = call "Texte in VIs uebersetzen.vi"("Sprachliste"=w197, "String zum Übersetzen"="Fehler beim Exportieren des .dbc Files" ("String")) -> ("String zum Übersetzen"=w198:string)  [unwired: 9 in, 4 out]
                n142 = One Button Dialog(message=w198) -> ()  [unwired: 1 in, 1 out]
              }
            }
          }
          frame True {
            n143 = One Button Dialog(message="Ungültiger Dateiname, muss auf .dbc enden !" ("Nachricht")) -> ()  [unwired: 1 in, 1 out]
          }
        }
      }
      event "Hinzufügen FTIR 1": Value Change {
        n144 = event-data() -> ()  [unwired: 1 in, 2 out]
        n145 = Unbundle By Name(w209) -> ("FTIR 1 Index"=w210:i32[])
        n146 = Build Array (concatenate)(w210, "Original Liste") -> (w202:i32[])
        n147 = for {
          tunnel: w202 -> [w213] mode=indexing
          tunnel: [w212] -> w205 mode=indexing
          tunnel: w204 -> [w211]
          n148 = Index Array(array=w211, index=w213) -> (element=w212:T10)
        }
        n149 = Bundle By Name(cluster=w209, "FTIR 1 Index"=w202) -> (w208:T9)
        n150 = property on="Konfigurierte Liste 1" class="Listenfeld (strikt)"("Item Names"=w205) -> (error out=w207:errorcluster)  [unwired: 2 in, 1 out]
        n151 = call <vilib>:"Clear Errors.vi"("error in (no error)"=w207) -> ()  [unwired: 5 in, 2 out]
      }
      event "Hinzufügen Status": Value Change {
        n152 = event-data() -> ()  [unwired: 1 in, 1 out]
        n153 = Unbundle By Name(w221) -> ("Status Index"=w222:i32[])
        n154 = Build Array (concatenate)(w222, "Statusliste") -> (w214:i32[])
        n155 = for {
          tunnel: w214 -> [w225] mode=indexing
          tunnel: [w224] -> w216 mode=indexing
          tunnel: w215 -> [w223]
          n156 = Index Array(array=w223, index=w225) -> (element=w224:T10)
        }
        n157 = Bundle By Name(cluster=w221, "Status Index"=w214) -> (w220:T9)
        n158 = property on="Konfigurierte Liste Status" class="Listenfeld (strikt)"("Item Names"=w216) -> (error out=w219:errorcluster)  [unwired: 2 in, 1 out]
        n159 = call <vilib>:"Clear Errors.vi"("error in (no error)"=w219) -> ()  [unwired: 5 in, 2 out]
      }
      event "Entfernen FTIR 1": Value Change {
        n160 = event-data() -> ()  [unwired: 1 in, 1 out]
        n161 = Unbundle By Name(w234) -> ("FTIR 1 Index"=w233:i32[])
        n162 = Delete From Array(array=w233, index="Konfigurierte Liste 1") -> (array with subset deleted=w228:i32[])  [unwired: 1 in, 1 out]
        n163 = for {
          tunnel: w228 -> [w237] mode=indexing
          tunnel: [w236] -> w226 mode=indexing
          tunnel: w227 -> [w235]
          n164 = Index Array(array=w235, index=w237) -> (element=w236:T10)
        }
        n165 = Bundle By Name(cluster=w234, "FTIR 1 Index"=w228) -> (w231:T9)
        n166 = property on="Konfigurierte Liste 1" class="Listenfeld (strikt)"("Item Names"=w226) -> (error out=w230:errorcluster)  [unwired: 2 in, 1 out]
        n167 = call <vilib>:"Clear Errors.vi"("error in (no error)"=w230) -> ()  [unwired: 5 in, 2 out]
      }
      event "Entfernen Status": Value Change {
        n168 = event-data() -> ()  [unwired: 1 in, 1 out]
        n169 = Unbundle By Name(w246) -> ("Status Index"=w245:i32[])
        n170 = Delete From Array(array=w245, index="Konfigurierte Liste Status") -> (array with subset deleted=w238:i32[])  [unwired: 1 in, 1 out]
        n171 = for {
          tunnel: w238 -> [w249] mode=indexing
          tunnel: [w248] -> w240 mode=indexing
          tunnel: w239 -> [w247]
          n172 = Index Array(array=w247, index=w249) -> (element=w248:T10)
        }
        n173 = Bundle By Name(cluster=w246, "Status Index"=w238) -> (w244:T9)
        n174 = property on="Konfigurierte Liste Status" class="Listenfeld (strikt)"("Item Names"=w240) -> (error out=w243:errorcluster)  [unwired: 2 in, 1 out]
        n175 = call <vilib>:"Clear Errors.vi"("error in (no error)"=w243) -> ()  [unwired: 5 in, 2 out]
      }
      event "Löschen FTIR 1": Value Change {
        n176 = event-data() -> ()  [unwired: 1 in, 1 out]
        n177 = Bundle By Name(cluster=w255, "FTIR 1 Index"=i32[] []) -> (w254:T9)
        n178 = property on="Konfigurierte Liste 1" class="Listenfeld (strikt)"("Item Names"=string[] [] ("Objektnamen")) -> (error out=w252:errorcluster)  [unwired: 2 in, 1 out]
        n179 = call <vilib>:"Clear Errors.vi"("error in (no error)"=w252) -> ()  [unwired: 5 in, 2 out]
      }
      event "Löschen Status": Value Change {
        n180 = event-data() -> ()  [unwired: 1 in, 1 out]
        n181 = Bundle By Name(cluster=w262, "Status Index"=i32[] [] ("FTIR 1 Index")) -> (w261:T9)
        n182 = property on="Konfigurierte Liste Status" class="Listenfeld (strikt)"("Item Names"=T10[] [] ("FTIR 1 Name")) -> (error out=w258:errorcluster)  [unwired: 2 in, 1 out]
        n183 = call <vilib>:"Clear Errors.vi"("error in (no error)"=w258) -> ()  [unwired: 5 in, 2 out]
      }
      event "Konfigurierte Liste 1": Drag Ended {
        n184 = event-data() -> ()  [unwired: 1 in, 5 out]
        n185 = property on="Konfigurierte Liste 1" class="Listenfeld (strikt)"() -> (error out=w271:errorcluster, "Item Names"=w272:string[])  [unwired: 2 in, 1 out]
        n186 = Unbundle By Name(w270) -> ("FTIR 1 Index"=w269:i32[], "FT-IR Scale"=w268:sgl[])
        n187 = call <vilib>:"Clear Errors.vi"("error in (no error)"=w271) -> ()  [unwired: 5 in, 2 out]
        n188 = local read "Optionsfelder FT-IR"() -> (w265:T4)
        n189 = for {
          tunnel: w274 -> [w293]
          tunnel: w272 -> [w292] mode=indexing
          tunnel: [w291] -> w267 mode=indexing
          n190 = Search 1D Array(1D array=w293, element=w292) -> (index of element=w291:i32)  [unwired: 1 in]
        }
        n191 = case shown="\"Optionsauswahl 2\"" w265 {
          tunnel: w267 -> [_ w283]
          tunnel: w269 -> [_ w282]
          tunnel: w268 -> [w275 w281]
          tunnel: [w275 w277] -> w266
          frame "Optionsauswahl 1", Default {
          }
          frame "Optionsauswahl 2" {
            n192 = for {
              tunnel: w283 -> [w289] mode=indexing
              tunnel: w282 -> [w290]
              tunnel: w281 -> [w287]
              shift-right: [w286] -> w277
              shift-left: sgl[] [] -> [w284]
              n193 = Search 1D Array(1D array=w290, element=w289) -> (index of element=w288:i32)  [unwired: 1 in]
              n194 = Delete From Array(array=w287, index=w288) -> (deleted portion=w285:sgl)  [unwired: 1 in, 1 out]
              n195 = Build Array (concatenate)(w284, w285) -> (w286:sgl[])
            }
            n196 = Number To Fractional String(number=w277) -> (F-format string=w279:string[])  [unwired: 3 in]
            n197 = Build Array(w279) -> (w278:string[][])
            n198 = Transpose 2D Array(2D array=w278) -> (transposed array=w276:string[][])
            n199 = local write "Tabellenelement FT-IR"(w276) -> ()
          }
        }
        n200 = Bundle By Name(cluster=w270, "FTIR 1 Index"=w267, "FT-IR Scale"=w266) -> (w273:T9)
      }
      event "Konfigurierte Liste Status": Drag Ended {
        n201 = event-data() -> ()  [unwired: 1 in, 5 out]
        n202 = Unbundle By Name(w300) -> ("Status Index"=w298:i32[], "Status Scale"=w297:sgl[])
        n203 = property on="Konfigurierte Liste Status" class="Listenfeld (strikt)"() -> (error out=w301:errorcluster, "Item Names"=w302:string[])  [unwired: 2 in, 1 out]
        n204 = local read "Optionsfelder Status"() -> (w296:T4)
        n205 = call <vilib>:"Clear Errors.vi"("error in (no error)"=w301) -> ()  [unwired: 5 in, 2 out]
        n206 = for {
          tunnel: w304 -> [w323]
          tunnel: w302 -> [w322] mode=indexing
          tunnel: [w321] -> w299 mode=indexing
          n207 = Search 1D Array(1D array=w323, element=w322) -> (index of element=w321:i32)  [unwired: 1 in]
        }
        n208 = case shown="\"Optionsauswahl 2\"" w296 {
          tunnel: w299 -> [_ w313]
          tunnel: w298 -> [_ w312]
          tunnel: w297 -> [w305 w311]
          tunnel: [w305 w306] -> w295
          frame "Optionsauswahl 1", Default {
          }
          frame "Optionsauswahl 2" {
            n209 = for {
              tunnel: w313 -> [w319] mode=indexing
              tunnel: w312 -> [w320]
              tunnel: w311 -> [w317]
              shift-right: [w316] -> w306
              shift-left: sgl[] [] -> [w314]
              n210 = Search 1D Array(1D array=w320, element=w319) -> (index of element=w318:i32)  [unwired: 1 in]
              n211 = Delete From Array(array=w317, index=w318) -> (deleted portion=w315:sgl)  [unwired: 1 in, 1 out]
              n212 = Build Array (concatenate)(w314, w315) -> (w316:sgl[])
            }
            n213 = Number To Fractional String(number=w306) -> (F-format string=w309:string[])  [unwired: 3 in]
            n214 = Build Array(w309) -> (w308:string[][])
            n215 = Transpose 2D Array(2D array=w308) -> (transposed array=w307:string[][])
            n216 = local write "Tabellenelement Status"(w307) -> ()
          }
        }
        n217 = Bundle By Name(cluster=w300, "Status Index"=w299, "Status Scale"=w295) -> (w303:T9)
      }
      event "Tabellenelement Status": Value Change {
        n218 = event-data() -> ()  [unwired: 1 in, 6 out]
        n219 = Fract/Exp String To Number(string="Tabellenelement Status", default (0 dbl)=sgl 0.0 ("Standard (0 DBL)")) -> (number=w329:sgl[][])  [unwired: 2 in, 1 out]
        n220 = Number To Fractional String(number=w329) -> (F-format string=w332:string[][])  [unwired: 3 in]
        n221 = Index Array(array=w329, index (col)=0 ("Deaktivierter Index (Spalte)")) -> (element=w326:sgl[])  [unwired: 1 in]
        n222 = local write "Tabellenelement Status"(w332) -> ()
        n223 = Bundle By Name(cluster=w327, "Status Scale"=w326) -> (w325:T9)
      }
      event "Tabellenelement FT-IR": Value Change {
        n224 = event-data() -> ()  [unwired: 1 in, 6 out]
        n225 = Fract/Exp String To Number(string="Tabellenelement FT-IR", default (0 dbl)=sgl 0.0 ("Standard (0 DBL)")) -> (number=w339:sgl[][])  [unwired: 2 in, 1 out]
        n226 = Number To Fractional String(number=w339) -> (F-format string=w342:string[][])  [unwired: 3 in]
        n227 = Index Array(array=w339, index (col)=0 ("Deaktivierter Index (Spalte)")) -> (element=w336:sgl[])  [unwired: 1 in]
        n228 = local write "Tabellenelement FT-IR"(w342) -> ()
        n229 = Bundle By Name(cluster=w337, "FT-IR Scale"=w336) -> (w335:T9)
      }
      event "Optionsfelder Status": Value Change {
        n230 = event-data() -> ()  [unwired: 1 in, 1 out]
        n231 = To Long Integer(number="Optionsfelder Status") -> (32bit integer=w346:i32)
        n232 = Bundle By Name(cluster=w348, "Optionsfelder Status"=w346) -> (w345:T9)
        n233 = case shown="\"Optionsauswahl 3\"" "Optionsfelder Status" {
          frame "Optionsauswahl 1", Default {
            n234 = property on="Tabellenelement Status" class="Tbl (strikt)"("Number of Rows"=u32 1 ("Zeilenanzahl")) -> ()  [unwired: 2 in, 2 out]
            n235 = property on="Tabellenelement Status" class="Tbl (strikt)"("Visible"=TRUE ("Sichtbar")) -> ()  [unwired: 2 in, 2 out]
          }
          frame "Optionsauswahl 2" {
            n236 = property on="Tabellenelement Status" class="Tbl (strikt)"("Number of Rows"=u32 8 ("Zeilenanzahl")) -> ()  [unwired: 2 in, 2 out]
            n237 = property on="Tabellenelement Status" class="Tbl (strikt)"("Visible"=TRUE ("Sichtbar")) -> ()  [unwired: 2 in, 2 out]
          }
          frame "Optionsauswahl 3" {
            n238 = property on="Tabellenelement Status" class="Tbl (strikt)"("Visible"=FALSE ("Sichtbar")) -> ()  [unwired: 2 in, 2 out]
          }
        }
      }
      event "Optionsfelder FT-IR": Value Change {
        n239 = event-data() -> ()  [unwired: 1 in, 1 out]
        n240 = To Long Integer(number="Optionsfelder FT-IR") -> (32bit integer=w357:i32)
        n241 = Bundle By Name(cluster=w359, "Optionsfelder FT-IR"=w357) -> (w356:T9)
        n242 = case shown="\"Optionsauswahl 1\", Standard" "Optionsfelder FT-IR" {
          frame "Optionsauswahl 1", Default {
            n243 = property on="Tabellenelement FT-IR" class="Tbl (strikt)"("Number of Rows"=u32 1 ("Zeilenanzahl")) -> ()  [unwired: 2 in, 2 out]
            n244 = property on="Tabellenelement FT-IR" class="Tbl (strikt)"("Visible"=TRUE ("Sichtbar")) -> ()  [unwired: 2 in, 2 out]
          }
          frame "Optionsauswahl 2" {
            n245 = property on="Tabellenelement FT-IR" class="Tbl (strikt)"("Number of Rows"=u32 13 ("Zeilenanzahl")) -> ()  [unwired: 2 in, 2 out]
            n246 = property on="Tabellenelement FT-IR" class="Tbl (strikt)"("Visible"=TRUE ("Sichtbar")) -> ()  [unwired: 2 in, 2 out]
          }
          frame "Optionsauswahl 3" {
            n247 = property on="Tabellenelement FT-IR" class="Tbl (strikt)"("Visible"=FALSE ("Sichtbar")) -> ()  [unwired: 2 in, 2 out]
          }
        }
      }
    }
  }
